vi "SetName.vi"(8 "error in (no error)":errorcluster, 10 "Name":string, 11 "3D Object in":refnum<class "3D Object.lvclass">) -> (0 "error out":errorcluster, 3 "3D Object out":refnum<class "3D Object.lvclass">)   [LabVIEW 2015, in "3D Object.lvclass"]
uses:
  3D Object.lvclass
  3D Object.lvclass/3D Object.ctl
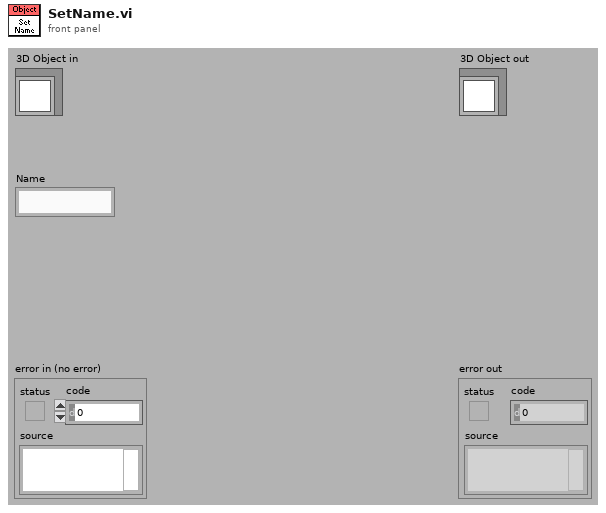
[diagram p1: front panel]
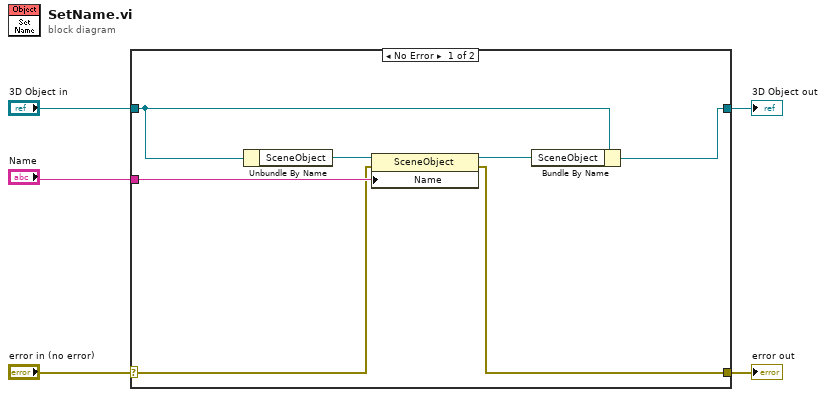
[diagram p0: block diagram]
diagram:
  n1 = case shown="No Error" "error in (no error)" {
    selector: "error in (no error)" -> [w7 w14]
    tunnel: [w6 w14] -> w4
    tunnel: [w9 w13] -> w2
    tunnel: "3D Object in" -> [w12 w13]
    tunnel: "Name" -> [w8 _]
    frame No Error {
      n2 = Unbundle By Name(w12) -> ("SceneObject"=w11:refnum<vi>)
      n3 = property class="SceneObject"(reference=w11, error in=w7, "Name"=w8) -> (reference out=w10:refnum<vi>, error out=w6:errorcluster)
      n4 = Bundle By Name(cluster=w12, "SceneObject"=w10) -> (w9:refnum<class "3D Object.lvclass">)
    }
    frame Error {
    }
  }
  "error out" <- w4
  "3D Object out" <- w2
